vi "Get 1 Algorithm Info.vi"(6 "Backend engine":T1, 8 "error in (no error)":errorcluster, 11 "Algorithm ID":string) -> (0 "error out":errorcluster, 3 "Algorithm Information":T2)   [LabVIEW 2013, in "QWTBLVLib.lvlib"]
doc: "Get informations of selected Algorithm."
uses:
  QWTBLVLib.lvlib
  TD Algorithm Information.ctl
  TD Algorithm Information Input.ctl
  TD Algorithm Information Output.ctl
  TD Backend Engine.ctl
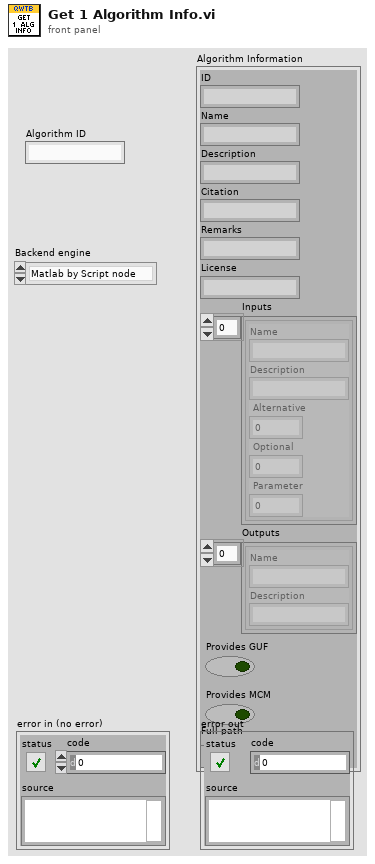
[diagram p1: front panel]
types:
  T1 = typedef "QWTBLVLib.lvlib/TD Backend Engine.ctl" = enum16{"Matlab by Script node", "GNU Octave by GOLPI"}
  T2 = typedef "QWTBLVLib.lvlib/TD Algorithm Information.ctl" = cluster{"ID":string, "Name":string, "Description":string, "Citation":string, "Remarks":string, "License":string, "Inputs":T3[], "Outputs":T4[], "Provides GUF":bool, "Provides MCM":bool, "Full path":string}
  T3 = typedef "QWTBLVLib.lvlib/TD Algorithm Information Input.ctl" = cluster{"Name":string, "Description":string, "Alternative":i32, "Optional":i32, "Parameter":i32}
  T4 = typedef "QWTBLVLib.lvlib/TD Algorithm Information Output.ctl" = cluster{"Name":string, "Description":string}
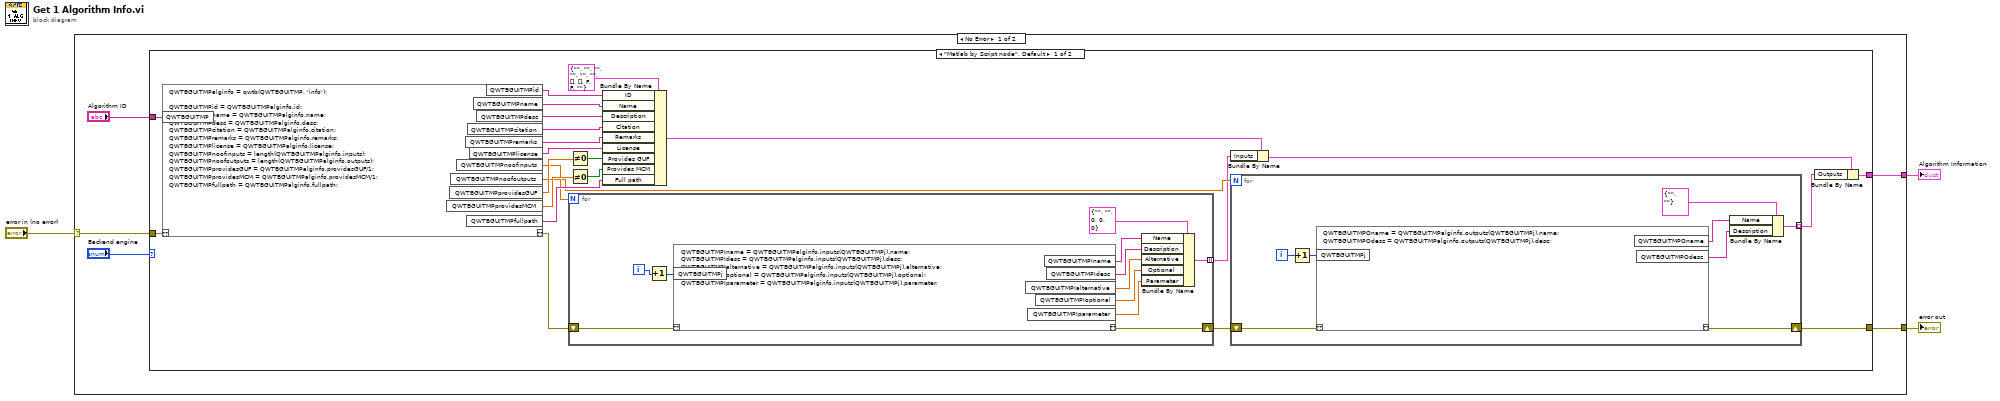
[diagram p0: block diagram]
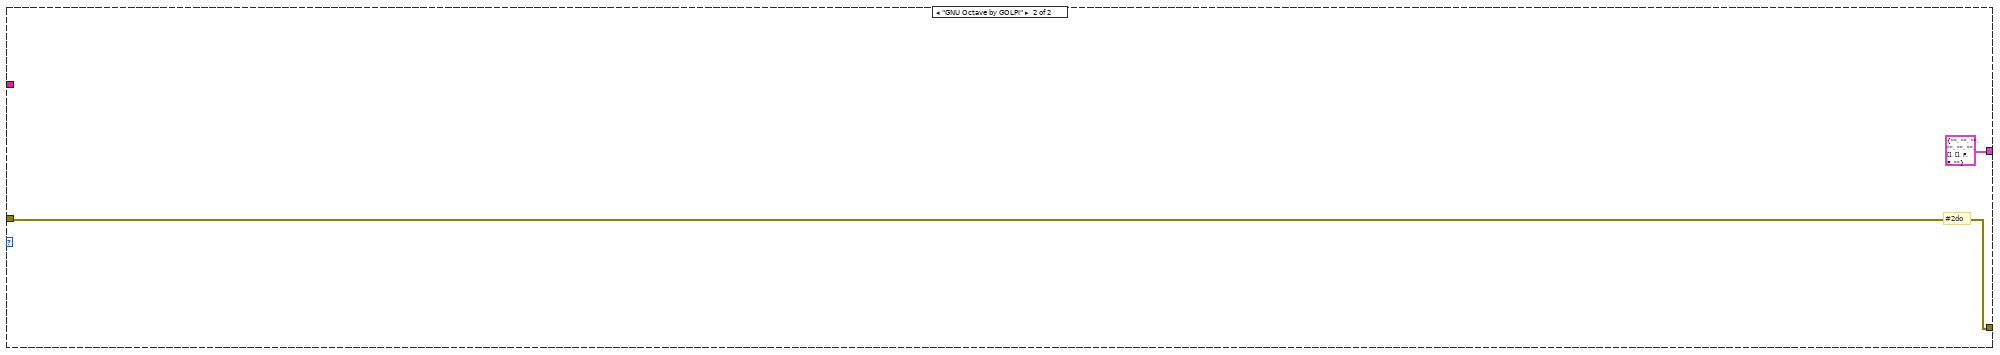
[diagram p2: hidden frame]
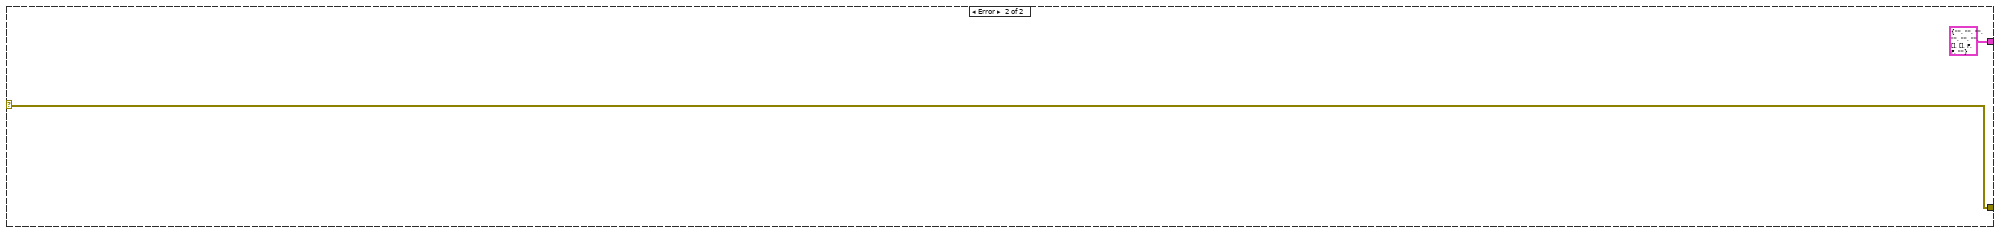
[diagram p3: hidden frame]
diagram:
  n1 = case shown="No Error" "error in (no error)" {
    selector: "error in (no error)" -> [w5 w54]
    tunnel: [w7 w54] -> w3
    tunnel: [w6 T2 {"ID"="", "Name"="", "Description"="", "Citation"="", "Remarks"="", "License"="", "Inputs"=[], "Outputs"=[], "Provides GUF"=FALSE, "Provides MCM"=FALSE, "Full path"=""} ("Algorithm Information")] -> w2
    frame No Error {
      n2 = case shown="\"Matlab by Script node\", Default" "Backend engine" {
        tunnel: "Algorithm ID" -> [w16 _]
        tunnel: [w13 w52] -> w7
        tunnel: [w12 T2 {"ID"="", "Name"="", "Description"="", "Citation"="", "Remarks"="", "License"="", "Inputs"=[], "Outputs"=[], "Provides GUF"=FALSE, "Provides MCM"=FALSE, "Full path"=""} ("Algorithm Information")] -> w6
        tunnel: w5 -> [w11 w52]
        frame "Matlab by Script node", Default {
          n3 = script code="QWTBGUITMPalginfo = qwtb(QWTBGUITMP, 'info');\n\nQWTBGUITMPid = QWTBGUITMPalginfo.id;\nQWTBGUITMPname = QWTBGUITMPalginfo.name;\nQWTBGUITMPdesc = QWTBGUITMPalginfo.desc;\nQWTBGUITMPcitation = QWTBGUITMPalginfo.citation;\nQWTBGUITMPremarks = QWTBGUITMPalginfo.remarks;\nQWTBGUITMPlicense = QWTBGUITMPalginfo.license;\nQWTBGUITMPnoofinputs = length(QWTBGUITMPalginfo.inputs);\nQWTBGUITMPnoofoutputs = length(QWTBGUITMPalginfo.outputs);\nQWTBGUITMPprovidesGUF = QWTBGUITMPalginfo.providesGUF/1;\nQWTBGUITMPprovidesMCM = QWTBGUITMPalginfo.providesMCM/1;\nQWTBGUITMPfullpath = QWTBGUITMPalginfo.fullpath;"("??"=w11, "QWTBGUITMP"=w16) -> ("??"=w20:errorcluster, "QWTBGUITMPid"=w30:string, "QWTBGUITMPname"=w29:string, "QWTBGUITMPdesc"=w28:string, "QWTBGUITMPfullpath"=w27:string, "QWTBGUITMPnoofinputs"=w19:dbl, "QWTBGUITMPnoofoutputs"=w17:dbl, "QWTBGUITMPcitation"=w21:string, "QWTBGUITMPremarks"=w22:string, "QWTBGUITMPprovidesGUF"=w24:dbl, "QWTBGUITMPprovidesMCM"=w26:dbl, "QWTBGUITMPlicense"=w32:string)
          n4 = for {
            N: w19 -> [_]
            shift-right: [w48] -> w18
            shift-left: w20 -> [w51]
            tunnel: [w46] -> w10 mode=indexing
            i -> [w49]
            n5 = Increment(x=w49) -> (x+1=w50:i32)
            n6 = script code="QWTBGUITMPIname = QWTBGUITMPalginfo.inputs(QWTBGUITMPj).name;\nQWTBGUITMPIdesc = QWTBGUITMPalginfo.inputs(QWTBGUITMPj).desc;\nQWTBGUITMPIalternative = QWTBGUITMPalginfo.inputs(QWTBGUITMPj).alternative;\nQWTBGUITMPIoptional = QWTBGUITMPalginfo.inputs(QWTBGUITMPj).optional;\nQWTBGUITMPIparameter = QWTBGUITMPalginfo.inputs(QWTBGUITMPj).parameter;"("??"=w51, "QWTBGUITMPj"=w50) -> ("??"=w48:errorcluster, "QWTBGUITMPIname"=w45:string, "QWTBGUITMPIdesc"=w44:string, "QWTBGUITMPIalternative"=w43:dbl, "QWTBGUITMPIoptional"=w42:dbl, "QWTBGUITMPIparameter"=w41:dbl)
            n7 = Bundle By Name(cluster=T3 {"Name"="", "Description"="", "Alternative"=0, "Optional"=0, "Parameter"=0} ("Algorithm Information Input"), "Name"=w45, "Description"=w44, "Alternative"=w43, "Optional"=w42, "Parameter"=w41) -> (w46:T3)
          }
          n8 = Not Equal To 0?(x=w24) -> (x != 0?=w23:bool)
          n9 = Not Equal To 0?(x=w26) -> (x != 0?=w25:bool)
          n10 = Bundle By Name(cluster=T2 {"ID"="", "Name"="", "Description"="", "Citation"="", "Remarks"="", "License"="", "Inputs"=[], "Outputs"=[], "Provides GUF"=FALSE, "Provides MCM"=FALSE, "Full path"=""} ("Algorithm Information"), "ID"=w30, "Name"=w29, "Description"=w28, "Citation"=w21, "Remarks"=w22, "License"=w32, "Provides GUF"=w23, "Provides MCM"=w25, "Full path"=w27) -> (w15:T2)
          n11 = Bundle By Name(cluster=w15, "Inputs"=w10) -> (w14:T2)
          n12 = for {
            N: w17 -> [_]
            shift-right: [w37] -> w13
            shift-left: w18 -> [w40]
            tunnel: [w35] -> w9 mode=indexing
            i -> [w38]
            n13 = Increment(x=w38) -> (x+1=w39:i32)
            n14 = script code="QWTBGUITMPOname = QWTBGUITMPalginfo.outputs(QWTBGUITMPj).name;\nQWTBGUITMPOdesc = QWTBGUITMPalginfo.outputs(QWTBGUITMPj).desc;"("??"=w40, "QWTBGUITMPj"=w39) -> ("??"=w37:errorcluster, "QWTBGUITMPOname"=w33:string, "QWTBGUITMPOdesc"=w34:string)
            n15 = Bundle By Name(cluster=T4 {"Name"="", "Description"=""} ("Algorithm Information Output"), "Name"=w33, "Description"=w34) -> (w35:T4)
          }
          n16 = Bundle By Name(cluster=w14, "Outputs"=w9) -> (w12:T2)
        }
        frame "GNU Octave by GOLPI" {
          # "#2do"
        }
      }
    }
    frame Error {
    }
  }
  "error out" <- w3
  "Algorithm Information" <- w2
